vi "fir_filterbank_test.vi"() -> ()   [LabVIEW 2013]
uses:
  <vilib>/measure/maspectr.llb/Power Spectrum and PSD Export Mode.ctl
  <vilib>/measure/maspectr.llb/FFT Power Spectrum and PSD for 1 Chan.vi
  <vilib>/measure/NI_MABase.lvlib
  <vilib>/measure/NI_MAPro.lvlib
panel:
  out "Waveform Graph out":dbl[](graph)
  out "Power spectrum in":cluster{"f0":dbl, "df":dbl, "magnitude":dbl[]}(graph)
  out "Power spectrum":cluster{"f0":dbl, "df":dbl, "magnitude":dbl[]}(graph)
  out "Waveform Graph":dbl[](graph)
  out "# of Iterations":i32
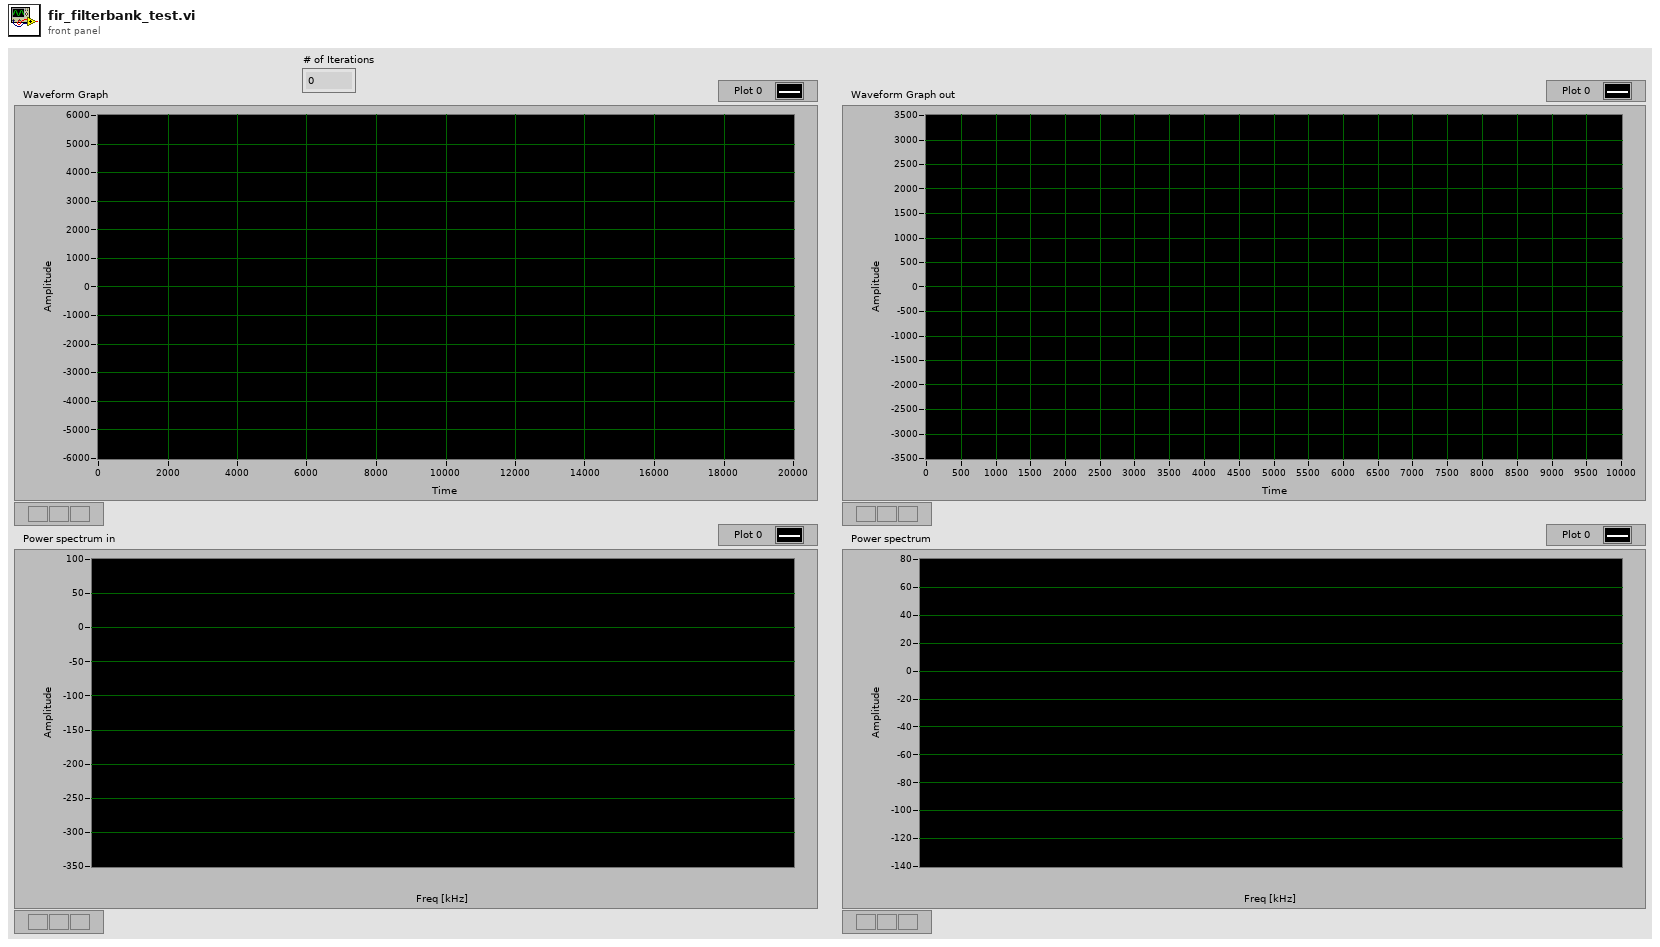
[diagram p1: front panel]
types:
  T1 = typedef "NI_MAPro.lvlib/Power Spectrum and PSD Export Mode.ctl" = u16
  T2 = cluster{"frequency":dbl, "amplitude":dbl, "phase":dbl}[]
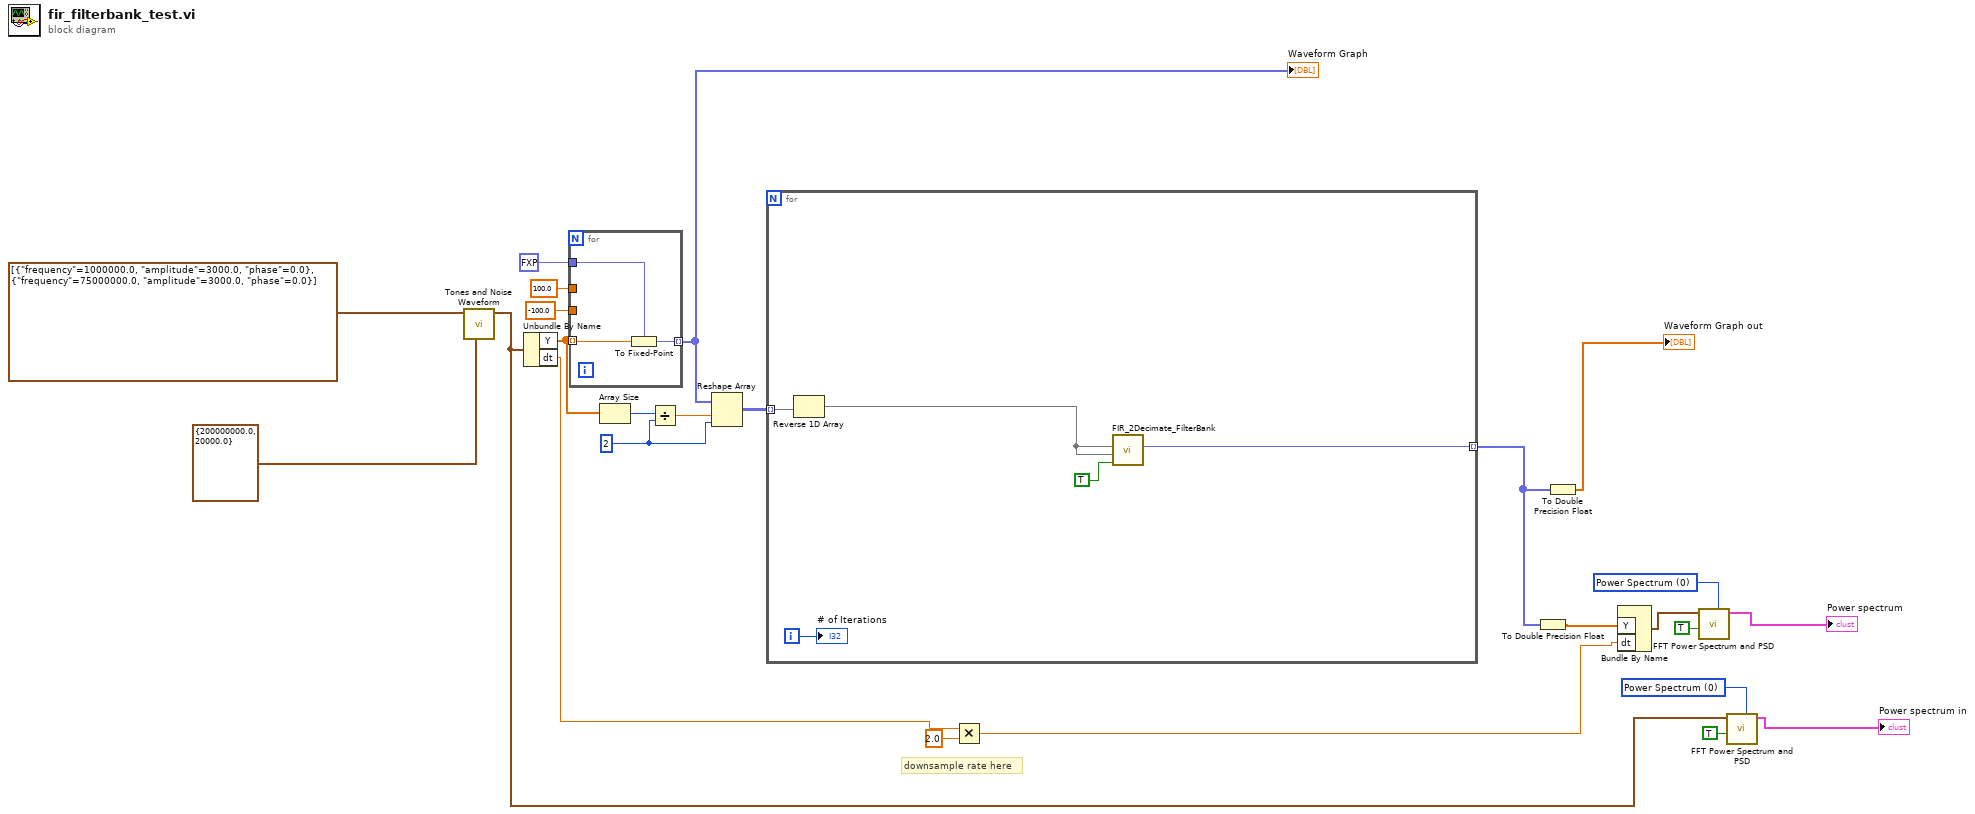
[diagram p0: block diagram]
diagram:
  w3 = 2 ("dimension size")
  w13 = T1 0 items=["Power Spectrum", "Power Spectral Density"] ("export mode")
  w21 = T1 0 items=["Power Spectrum", "Power Spectral Density"] ("export mode")
  # "downsample rate here"
  n1 = call <vilib>:"Tones and Noise Waveform.vi"("sampling info"=cluster{"Fs":dbl, "#s":dbl} {"Fs"=200000000.0, "#s"=20000.0}, "tones"=T2 [{"frequency"=1000000.0, "amplitude"=3000.0, "phase"=0.0}, {"frequency"=75000000.0, "amplitude"=3000.0, "phase"=0.0}]) -> ("signal out"=w12:waveform(dbl))  [unwired: 8 in, 1 out]
  n2 = Unbundle By Name(w12) -> ("Y"=w6:dbl[], "dt"=w19:dbl)
  n3 = for {
    tunnel: w6 -> [w27] mode=indexing
    tunnel: fxp<+/-,16,14> 0.0 ("fixed-point type") -> [w28]
    tunnel: [w26] -> w2 mode=indexing
    tunnel: 100.0 -> [_]
    tunnel: -100.0 -> [_]
    n4 = To Fixed-Point(fixed-point type=w28, number=w27) -> (fixed-point=w26:fxp<+/-,16,14>)
  }
  "Waveform Graph" <- w2
  n5 = Array Size(array=w6) -> (size(s)=w5:i32)
  n6 = Divide(x=w5, y=w3) -> (x/y=w4:dbl)
  n7 = Reshape Array(w2, w4, w3) -> (w1:fxp<+/-,16,14>[][])
  n8 = for {
    tunnel: [w31] -> w7 mode=indexing
    tunnel: w1 -> [w30] mode=indexing
    i -> [w33]
    n9 = Reverse 1D Array(array=w30) -> (reversed array=w29:fxp<+/-,16,14>[])
    n10 = call "FIR_2Decimate_FilterBank.vi"("data valid in"=TRUE, "Q in"=w29, "I in"=w29) -> ("I out"=w31:fxp<+/-,16,14>)  [unwired: 6 in, 2 out]
    "# of Iterations" <- w33
  }
  n11 = Multiply(x=w19, y=2.0) -> (x*y=w17:dbl)
  n12 = To Double Precision Float(number=w7) -> (double precision float=w15:dbl[])
  n13 = To Double Precision Float(number=w7) -> (double precision float=→"Waveform Graph out":dbl[])
  n14 = Bundle By Name("Y"=w15, "dt"=w17) -> (w22:waveform(dbl))  [unwired: 1 in]
  n15 = call-poly <vilib>:"FFT Power Spectrum and PSD.vi"("export mode"=w21, "dB On (F)"=TRUE, "time signal"=w22) -> ("Power Spectrum / PSD"=→"Power spectrum":cluster{"f0":dbl, "df":dbl, "magnitude":dbl[]})  [unwired: 5 in, 3 out]
  n16 = call-poly <vilib>:"FFT Power Spectrum and PSD.vi"("export mode"=w13, "dB On (F)"=TRUE, "time signal"=w12) -> ("Power Spectrum / PSD"=→"Power spectrum in":cluster{"f0":dbl, "df":dbl, "magnitude":dbl[]})  [unwired: 5 in, 3 out]
